vi "2022_day8_sub_calculate_1D_scenic_score.vi"(9 "Element Idx":i32, 10 "Array In":i32[](array[numeric])) -> (1 "Result":i32)   [LabVIEW 2021]
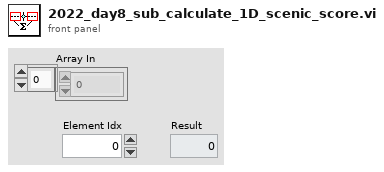
[diagram p1: front panel]
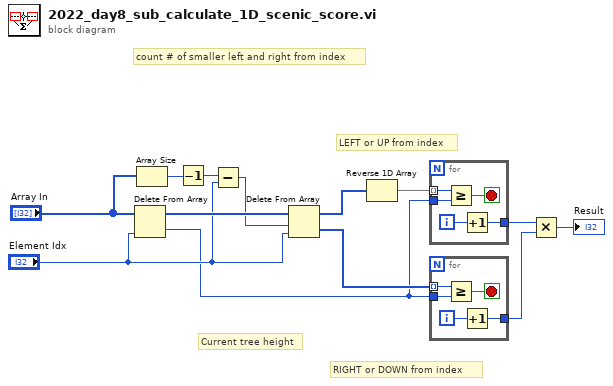
[diagram p0: block diagram]
diagram:
  # "Current tree height"
  # "RIGHT or DOWN from index"
  # "LEFT or UP from index"
  # "count # of smaller left and right from index"
  n1 = Delete From Array(array="Array In", index="Element Idx") -> (deleted portion=w4:i32, array with subset deleted=w13:i32[])  [unwired: 1 in]
  n2 = Array Size(array="Array In") -> (size(s)=w11:i32)
  n3 = Decrement(x=w11) -> (x-1=w10:i32)
  n4 = Subtract(x=w10, y="Element Idx") -> (x-y=w8:i32)
  n5 = Delete From Array(array=w13, length=w8, index="Element Idx") -> (deleted portion=w5:i32[], array with subset deleted=w7:i32[])
  n6 = Reverse 1D Array(array=w7) -> (reversed array=w6:i32[])
  n7 = for {
    tunnel: w6 -> [w18] mode=indexing
    tunnel: w4 -> [w17]
    tunnel: [w15] -> w3
    i -> [w16]
    stop <- w14 stop-if-true
    n8 = Greater Or Equal?(x=w18, y=w17) -> (x >= y?=w14:bool)
    n9 = Increment(x=w16) -> (x+1=w15:i32)
  }
  n10 = for {
    tunnel: w5 -> [w23] mode=indexing
    tunnel: w4 -> [w22]
    tunnel: [w20] -> w2
    i -> [w21]
    stop <- w19 stop-if-true
    n11 = Greater Or Equal?(x=w23, y=w22) -> (x >= y?=w19:bool)
    n12 = Increment(x=w21) -> (x+1=w20:i32)
  }
  n13 = Multiply(x=w3, y=w2) -> (x*y=→"Result":i32)
